vi "Memento.vi"(8 "error in (no error)":errorcluster, 10 "State":string, 11 "Memento in":refnum<class "Memento.lvclass">) -> (0 "error out":errorcluster, 3 "Memento out":refnum<class "Memento.lvclass">)   [LabVIEW 2017, in "Memento.lvclass"]
uses:
  Memento.lvclass
  Memento.lvclass/Memento.ctl
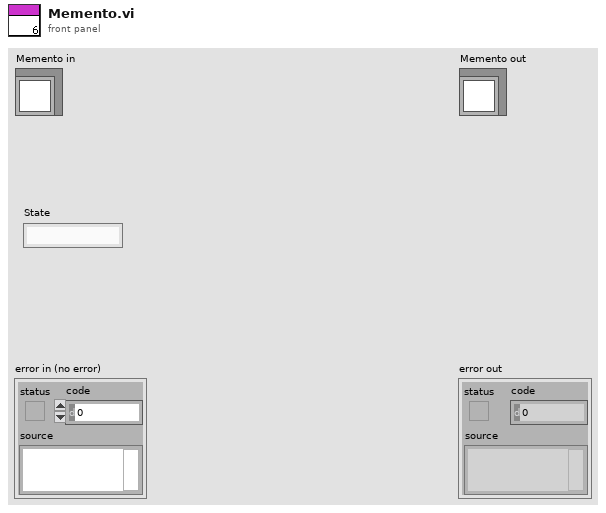
[diagram p1: front panel]
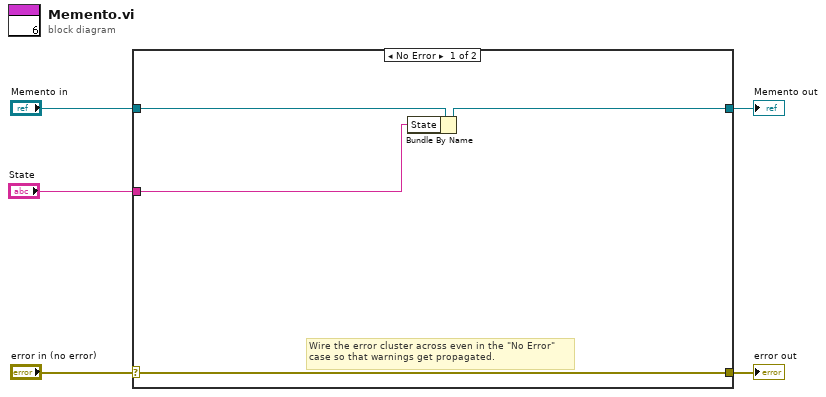
[diagram p0: block diagram]
diagram:
  n1 = case shown="No Error" "error in (no error)" {
    selector: "error in (no error)" -> [w8 w11]
    tunnel: [w8 w11] -> w4
    tunnel: [w7 w10] -> w2
    tunnel: "Memento in" -> [w9 w10]
    tunnel: "State" -> [w6 _]
    frame No Error {
      # "Wire the error cluster across even in the \"No Error\"\ncase so that warnings get propagated."
      n2 = Bundle By Name(cluster=w9, "State"=w6) -> (w7:refnum<class "Memento.lvclass">)
    }
    frame Error {
    }
  }
  "error out" <- w4
  "Memento out" <- w2
